vi "FPGA_main.vi"() -> ()   [LabVIEW 2018]
doc: "FPGA main VI for AI input and output.\n\nSamples at 100 kHz and downsamples to 1 kHz."
uses:
  <vilib>/rvi/Emulation/niFpgaGetClockAttributes.vi
  <vilib>/rvi/Emulation/niFpgaSctlEmulationGetInTimedLoop.vi
  <vilib>/rvi/Emulation/niFpgaEmulationReportErrorSimple.vi
  <vilib>/rvi/eio/common/nirviEmuTemplateMethod_errors.vi
  <vilib>/rvi/Emulation/niFpgaEmulationIsFPGAContextNoSignature.vi
  <vilib>/rvi/errors/niFpgaSetErrorForExecOnDevCompSimple.vi
  <vilib>/rvi/eio/common/nirviEmuReportErrorAndStop.vi
  <vilib>/rvi/DataTransferAndStorage/Container/Common/niFpgaContainerGetUniqueNameForEmu.vi
  <vilib>/rvi/FIFO/Fifo_Resource/nirvififoEmulationSetSize.vi
  <vilib>/rvi/FIFO/Fifo_Resource/nirviFifoEmulationQueueMgr.vi
  <instcachedir>/0/nirviFifoEmulationQueueMgr_E5CAEC123FF24DC58D834DCA3CDAA9B5.lvgen/nirviFifoEmulationQueueMgr_E5CAEC123FF24DC58D834DCA3CDAA9B5_003.vi
  <vilib>/rvi/FIFO/Fifo_Resource/nirvififoEmulationDetermineInputValidOut.vi
  <vilib>/rvi/FIFO/Fifo_Resource/nirvififoEmulationCreateLock.vi
  <vilib>/rvi/Emulation/niFpgaProcessEmulError.vi
  <vilib>/rvi/FIFO/Fifo_Resource/nirvififoEmulationObtainLock.vi
  <vilib>/rvi/FIFO/Fifo_Resource/nirvififoEmulationReleaseLock.vi
  <vilib>/rvi/occurrence/nirviWaitOnOccurrenceBase.vi
  <vilib>/rvi/errors/nirviReportUnexpectedCaseInternalError.vi
  <vilib>/rvi/errors/nirviReportUnexpectedCaseInternalError (U32).vi
  <vilib>/rvi/Emulation/niFpgaCriticalErrorInLSC.vi
  <vilib>/Utility/error.llb/Clear Errors.vi
  <vilib>/eio/EIONode/EIONode.xnode
  <vilib>/rvi/DataTransferAndStorage/Container/XNode/niFpgaContainer.xnode
  <vilib>/rvi/FIFO/Fifo_Resource/nirvififoEmulationWrite.vi
  <vilib>/rvi/Analysis/measure/butterworth/XNode/niFpgaButterworthFilter.xnode
  <vilib>/rvi/FIFO/Fifo_Resource/nirvififoEmulationRead.vi
panel:
  in  "Count(uSec)":u8=8 caption="I/O sample time (us)"
  out "LPF loop rate (us)":u8
  out "ConnectorC/AI1":fxp<+/-,20,20>
  out "ConnectorC/AI0":fxp<+/-,20,20>
  out "Signal I/O loop rate (us)":u8
  in  "ConnectorC/AO1":i16
  in  "ConnectorC/AO0":i16
  # "Inputs"
  # "Sampling time"
  # "Filtered AI"
  # "For each additional bit of resolution, the signal must be oversampled by a factor of four:\nf_os = 4^w f_s \nwhere w is the number of additional bits of resolution desired, f_s is the original sampling frequency requirement, and f_os is the oversampling frequency\n\nhttp://www.cypress.com/file/236481/download"
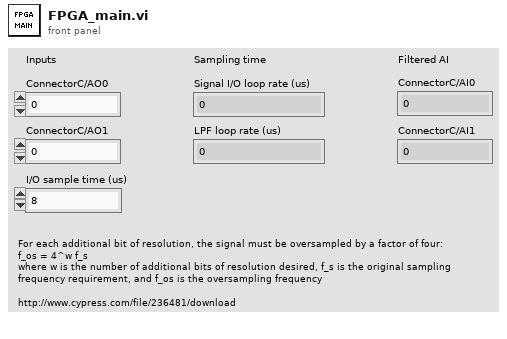
[diagram p1: front panel]
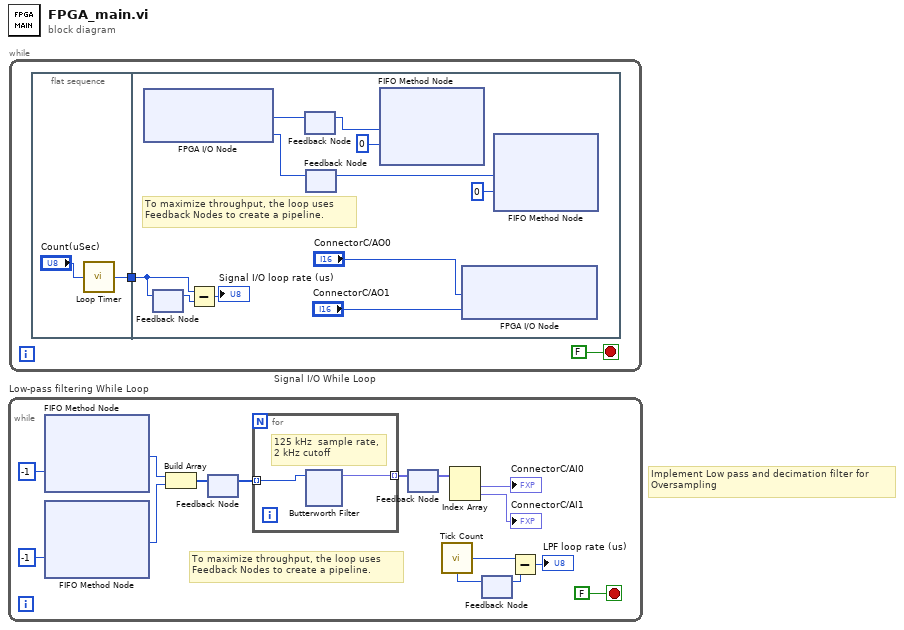
[diagram p0: block diagram]
diagram:
  # "Implement Low pass and decimation filter for \nOversampling"
  n1 = while "Low-pass filtering While Loop" {
    stop <- FALSE stop-if-true
    # "To maximize throughput, the loop uses \nFeedback Nodes to create a pipeline."
    n2 = xnode ("FIFO Method Node")("Timeout"=-1) -> ("Element"=w13:i16)  [unwired: 1 in, 2 out]
    n3 = xnode ("FIFO Method Node")("Timeout"=-1) -> ("Element"=w12:i16)  [unwired: 1 in, 2 out]
    n4 = Build Array(w13, w12) -> (w3:i16[])
    n5 = feedback-in #1(w3) -> ()
    n6 = feedback #1() -> (w4:i16[])  [unwired: 1 in]
    n7 = for {
      tunnel: w4 -> [w16] mode=indexing
      tunnel: [w15] -> w1 mode=indexing
      # "125 kHz  sample rate,\n2 kHz cutoff"
      n8 = xnode "Butterworth Filter"("input data"=w16) -> ("output data"=w15:fxp<+/-,20,20>)  [unwired: 2 in, 1 out]
    }
    n9 = feedback #2() -> (w2:fxp<+/-,20,20>[])  [unwired: 1 in]
    n10 = feedback-in #2(w1) -> ()
    n11 = call "Tick Count"() -> ("Tick Count(uSec)"=w7:u8)
    n12 = Index Array(array=w2) -> (element #1=→"ConnectorC/AI0":fxp<+/-,20,20>, element #2=→"ConnectorC/AI1":fxp<+/-,20,20>)  [unwired: 2 in]
    n13 = feedback-in #3(w7) -> ()
    n14 = feedback #3() -> (w6:u8)  [unwired: 1 in]
    n15 = Subtract(x=w7, y=w6) -> (x-y=→"LPF loop rate (us)":u8)
  }
  n16 = while "Signal I/O While Loop" {
    stop <- FALSE stop-if-true
    n17 = flat-sequence {
      tunnel: [w29] -> w26
      tunnel: w26 -> [w39]
      frame #0 {
        n18 = call "Loop Timer"("Count(uSec)"="Count(uSec)") -> ("Tick Count(uSec)"=w29:u8)
      }
      frame #1 {
        # "To maximize throughput, the loop uses \nFeedback Nodes to create a pipeline."
        n19 = xnode "FPGA I/O Node"() -> ("ConnectorC/AI0"=w37:i16, "ConnectorC/AI1"=w35:i16)  [unwired: 2 in, 2 out]
        n20 = feedback #4() -> (w40:u8)  [unwired: 1 in]
        n21 = feedback-in #4(w39) -> ()
        n22 = Subtract(x=w39, y=w40) -> (x-y=→"Signal I/O loop rate (us)":u8)
        n23 = feedback-in #5(w37) -> ()
        n24 = feedback #5() -> (w33:i16)  [unwired: 1 in]
        n25 = feedback-in #6(w35) -> ()
        n26 = feedback #6() -> (w32:i16)  [unwired: 1 in]
        n27 = xnode ("FIFO Method Node")("Element"=w33, "Timeout"=0) -> ()  [unwired: 1 in, 2 out]
        n28 = xnode "FPGA I/O Node"("ConnectorC/AO0"="ConnectorC/AO0", "ConnectorC/AO1"="ConnectorC/AO1") -> ()  [unwired: 2 in, 2 out]
        n29 = xnode ("FIFO Method Node")("Element"=w32, "Timeout"=0) -> ()  [unwired: 1 in, 2 out]
      }
    }
  }
